vi "Config Mode.vi"(0 "VISA resource name":refnum<visa-resource-name>, 5 "Mode (0: RMS)":u16(ring) items=["RMS", "V-MEAN", "DC"], 11 "error in (no error)":errorcluster) -> (4 "VISA resource name out":refnum<visa-resource-name>, 15 "error out":errorcluster)   [LabVIEW 2023, in "Yokogawa WT200 Series.lvlib"]
doc: "This VI sends the measurement mode command of current and voltage to the WT200 Series."
uses:
  Yokogawa WT200 Series.lvlib
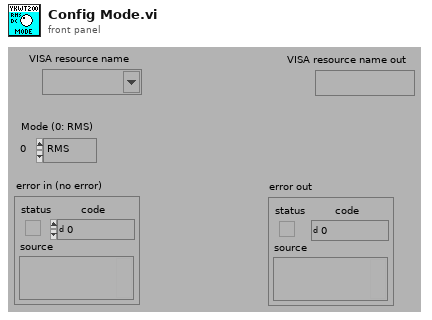
[diagram p1: front panel]
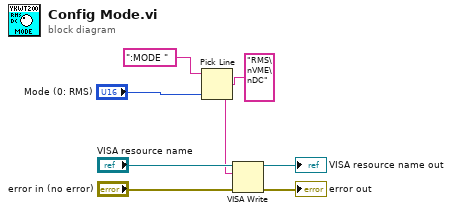
[diagram p0: block diagram]
diagram:
  n1 = Pick Line(string ("")=":MODE ", multi-line string="RMS\nVME\nDC", line index="Mode (0: RMS)") -> (output string=w1:string)
  n2 = VISA Write(VISA resource name="VISA resource name", write buffer=w1, error in (no error)="error in (no error)") -> (VISA resource name out=→"VISA resource name out":refnum<visa-resource-name>, error out=→"error out":errorcluster)  [unwired: 1 out]
